vi "mqttCmdSendReceive.vi"(0 "mqttConnect in":refnum<class "mqttCmd.lvclass">, 5 "byte1":u8, 11 "error in (no error)":errorcluster) -> (4 "mqttConnect out":refnum<class "mqttCmd.lvclass">, 8 "notification":T1, 15 "error out":errorcluster)   [LabVIEW 2015, in "mqttCmd.lvclass"]
uses:
  mqttCmd.lvclass
  mqttTypedef/mqttRXdataCluster.ctl
  mqttTypedef/mqttFixedHeaderResponse.ctl
  mqttTypedef/mqttQOSlevel.ctl
  mqttTypedef/mqttMessageType.ctl
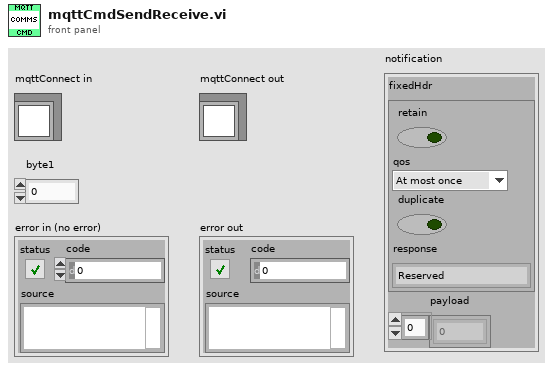
[diagram p1: front panel]
types:
  T1 = typedef "mqttRXdataCluster.ctl" = cluster{"fixedHdr":T2, "payload":u8[]}
  T2 = typedef "mqttFixedHeaderResponse.ctl" = cluster{"retain":bool, "qos":T3, "duplicate":bool, "response":T4}
  T3 = typedef "mqttQOSlevel.ctl" = enum8{"At most once", "At least once", "Exactly once", "Reserved"}
  T4 = typedef "mqttMessageType.ctl" = enum32{"Reserved", "CONNECT", "CONNACK", "PUBLISH", "PUBACK", "PUBREC", "PUBREL", "PUBCOMP", "SUBSCRIBE", "SUBACK", "UNSUBSCRIBE", "UNSUBACK", "PINGREQ", "PINGRESP", "DISCONNECT", "Reserved2"}
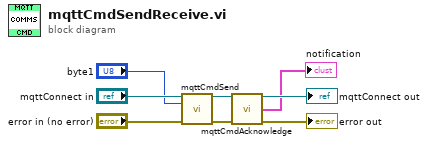
[diagram p0: block diagram]
diagram:
  n1 = call "mqttCmdSend.vi"("mqttBrokerCommand in"="mqttConnect in", "byte1"="byte1", "error in (no error)"="error in (no error)") -> ("mqttBrokerCommand out"=w5:refnum<class "mqttCmd.lvclass">, "error out"=w6:errorcluster)  [unwired: 11 in]
  n2 = call-dynamic "mqttCmdAcknowledge.vi"("_mqtt in"=w5, "error in (no error)"=w6) -> ("_mqtt out"=→"mqttConnect out":refnum<class "mqttCmd.lvclass">, "notification"=→"notification":T1, "error out"=→"error out":errorcluster)  [unwired: 11 in]
